vi "Add File Menu.vi"(8 "error in":errorcluster, 10 "File Info":T1, 11 "Menu Ref":refnum<k9>) -> (0 "error out":errorcluster)   [LabVIEW 2020, in "Peer Review.lvclass"]
uses:
  Peer Review.lvclass
  TypeDefs/File Info.ctl
  TypeDefs/File State.ctl
  TypeDefs/VI Type.ctl
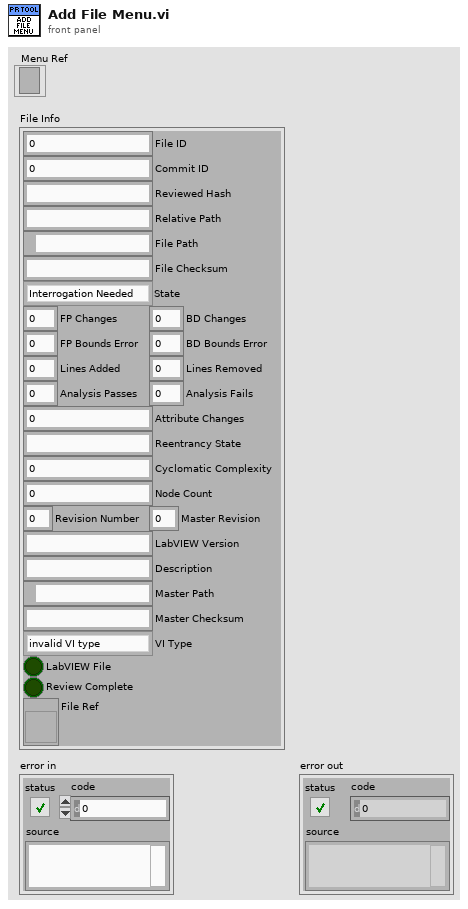
[diagram p1: front panel]
types:
  T1 = typedef "Peer Review.lvclass/File Info.ctl" = cluster{"File ID":i32, "Commit ID":i32, "Reviewed Hash":string, "Relative Path":string, "File Path":path, "File Checksum":string, "State":T2, "FP Changes":i32, "BD Changes":i32, "FP Bounds Error":dbl, "BD Bounds Error":dbl, "Lines Added":i32, "Lines Removed":i32, "Analysis Passes":i32, "Analysis Fails":i32, "Attribute Changes":i32, "Reentrancy State":string, "Cyclomatic Complexity":i32, "Node Count":i32, "Revision Number":u32, "LabVIEW Version":string, "Description":string, "Master Path":path, "Master Checksum":string, "VI Type":T3, "LabVIEW File":bool, "Review Complete":bool, "File Ref":refnum<vi>, "Master Revision":u32}
  T2 = typedef "Peer Review.lvclass/File State.ctl" = enum16{"Interrogation Needed", "Modified", "Deleted", "Added", "Matches Previous", "No Changes", "Moved", "Empty File"}
  T3 = typedef "Peer Review.lvclass/VI Type.ctl" = enum32{"invalid VI type", "Standard VI", "Control VI", "Global VI", "Polymorphic VI", "Configuration VI", "SubSystem", "Facade VI", "Method VI", "Statechart Diagram VI"}
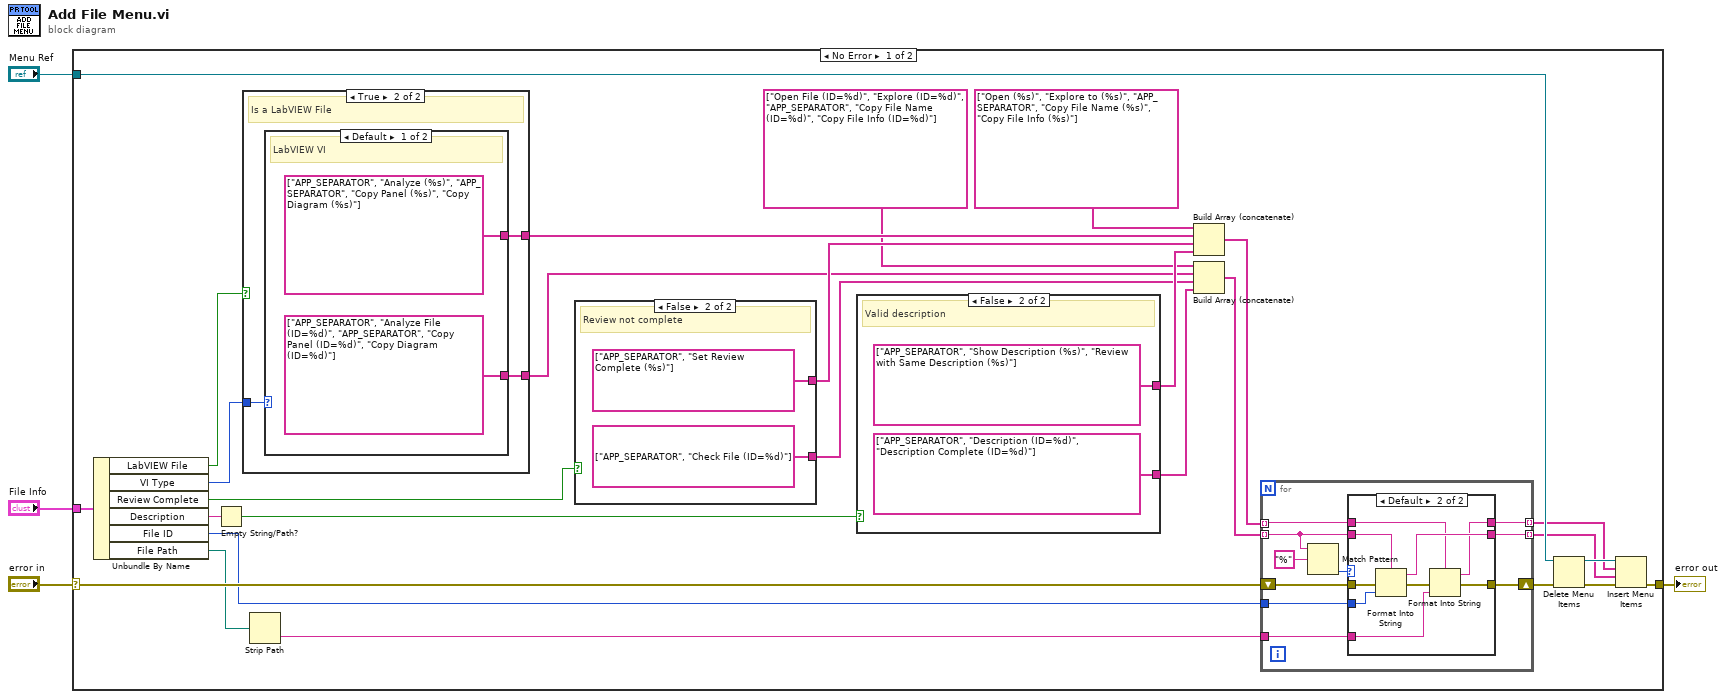
[diagram p0: block diagram]
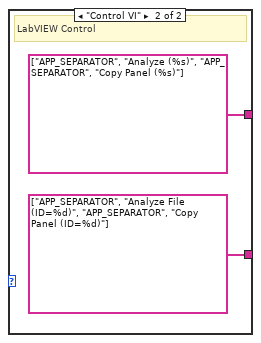
[diagram p3: hidden frame]
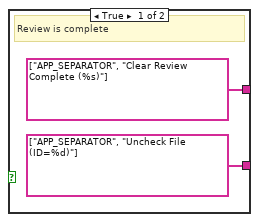
[diagram p5: hidden frame]
diagram:
  n1 = case shown="No Error" "error in" {
    selector: "error in" -> [w20 w67]
    tunnel: "File Info" -> [w17 _]
    tunnel: [w31 w67] -> w3
    tunnel: "Menu Ref" -> [w28 _]
    frame No Error {
      n2 = Unbundle By Name(w17) -> ("LabVIEW File"=w16:bool, "VI Type"=w15:T3, "Review Complete"=w21:bool, "Description"=w22:string, "File ID"=w18:i32, "File Path"=w19:path)
      n3 = Empty String/Path?(string/path=w22) -> (empty?=w23:bool)
      n4 = case shown="True" w16 {
        tunnel: [_ w34] -> w14
        tunnel: [_ w33] -> w9
        tunnel: w15 -> [_ w32]
        frame False {
          # "Is not a LabVIEW File"
        }
        frame True {
          # "Is a LabVIEW File"
          n5 = case shown="Default" w32 {
            tunnel: [string[] ["APP_SEPARATOR", "Analyze File (ID=%d)", "APP_SEPARATOR", "Copy Panel (ID=%d)", "Copy Diagram (ID=%d)"] ("format string") string[] ["APP_SEPARATOR", "Analyze File (ID=%d)", "APP_SEPARATOR", "Copy Panel (ID=%d)"] ("format string")] -> w33
            tunnel: [string[] ["APP_SEPARATOR", "Analyze (%s)", "APP_SEPARATOR", "Copy Panel (%s)", "Copy Diagram (%s)"] ("format string") string[] ["APP_SEPARATOR", "Analyze (%s)", "APP_SEPARATOR", "Copy Panel (%s)"] ("format string")] -> w34
            frame Default {
              # "LabVIEW VI"
            }
            frame "Control VI" {
              # "LabVIEW Control"
            }
          }
        }
      }
      n6 = Strip Path(path=w19) -> (name=w24:string)  [unwired: 1 out]
      n7 = case shown="False" w21 {
        tunnel: [string[] ["APP_SEPARATOR", "Clear Review Complete (%s)"] ("format string") string[] ["APP_SEPARATOR", "Set Review Complete (%s)"] ("format string")] -> w12
        tunnel: [string[] ["APP_SEPARATOR", "Uncheck File (ID=%d)"] ("format string") string[] ["APP_SEPARATOR", "Check File (ID=%d)"] ("format string")] -> w8
        frame True {
          # "Review is complete"
        }
        frame False {
          # "Review not complete"
        }
      }
      n8 = case shown="False" w23 {
        tunnel: [_ string[] ["APP_SEPARATOR", "Show Description (%s)", "Review with Same Description (%s)"] ("format string")] -> w13
        tunnel: [_ string[] ["APP_SEPARATOR", "Description (ID=%d)", "Description Complete (ID=%d)"] ("format string")] -> w7
        frame True {
          # "No description"
        }
        frame False {
          # "Valid description"
        }
      }
      n9 = Build Array (concatenate)(string[] ["Open (%s)", "Explore to (%s)", "APP_SEPARATOR", "Copy File Name (%s)", "Copy File Info (%s)"] ("format string"), w14, w12, w13) -> (w5:string[])
      n10 = Build Array (concatenate)(string[] ["Open File (ID=%d)", "Explore (ID=%d)", "APP_SEPARATOR", "Copy File Name (ID=%d)", "Copy File Info (ID=%d)"] ("format string"), w9, w8, w7) -> (w6:string[])
      n11 = for {
        tunnel: w18 -> [w54]
        tunnel: w6 -> [w46] mode=indexing
        shift-right: [w49] -> w29
        shift-left: w20 -> [w48]
        tunnel: [w53] -> w26 mode=indexing
        tunnel: w24 -> [w52]
        tunnel: w5 -> [w51] mode=indexing
        tunnel: [w50] -> w25 mode=indexing
        n12 = Match Pattern(string=w46, regular expression="%") -> (offset past match=w45:i32)  [unwired: 1 in, 3 out]
        n13 = case shown="Default" w45 {
          tunnel: w54 -> [_ w66]
          tunnel: [w56 w65] -> w53
          tunnel: w52 -> [_ w64]
          tunnel: w51 -> [w57 w63]
          tunnel: [w57 w62] -> w50
          tunnel: [w55 w60] -> w49
          tunnel: w48 -> [w55 w59]
          tunnel: w46 -> [w56 w58]
          frame -1 {
            # "For separator line"
          }
          frame Default {
            n14 = Format Into String(format string=w58, error in=w59, w66) -> (resulting string=w65:string, error out=w61:errorcluster)  [unwired: 1 in]
            n15 = Format Into String(format string=w63, error in=w61, w64) -> (resulting string=w62:string, error out=w60:errorcluster)  [unwired: 1 in]
          }
        }
      }
      n16 = Delete Menu Items(6:w29, 9:w28) -> (0:w30:errorcluster, 3:w27:refnum<k9>)  [unwired: 2 in]
      n17 = Insert Menu Items(6:w30, 7:w26, 8:w25, 9:w27) -> (0:w31:errorcluster)  [unwired: 2 in, 2 out]
    }
    frame Error {
    }
  }
  "error out" <- w3
